vi "DAQmx Device Name.vi"(1 "DAQmx Device Name":tag) -> (0 "DAQmx Device Name Out":tag)   [LabVIEW 2012]
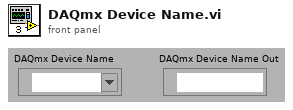
[diagram p1: front panel]
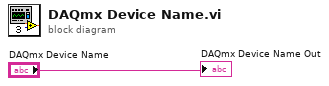
[diagram p0: block diagram]
diagram:
  "DAQmx Device Name Out" <- "DAQmx Device Name"
